vi "AFT Filter Signal (Real, PtByPt).vi"(7 "reset? (F)":bool, 8 "error in (no error)":errorcluster, 10 "x(n)":dbl, 11 "adaptive filter in":refnum<k20>) -> (0 "error out":errorcluster, 2 "y(n)":dbl, 3 "adaptive filter out":refnum<k20>)   [LabVIEW 2017, in "NI_AdaptiveFilter.lvlib"]
doc: "Filters an input signal with an adaptive filter point by point. You must use the least mean squares (LMS) or recursive least squares (RLS) algorithms to create the adaptive filter. Unlike the AFT Filter Signal and Update Coefficients VI, the AFT Filter Signal VI does not update the coefficients of the adaptive filter. Use the AFT Update Coefficients VI to update the filter coefficients. Wire data to the <B>x(n)</B> input to determine the polymorphic instance to use or manually select the instance. The data type of the adaptive filter that you wire to the <B>adaptive filter in</B> input must match the instance of the AFT Filter Signal VI."
uses:
  <vilib>/addons/Adaptive Filters/NI_AdaptiveFilter.lvlib
  <resource>/AdaptiveFilters.dll
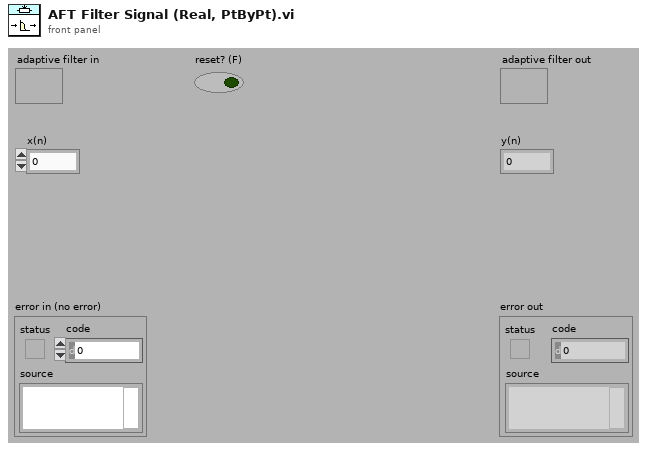
[diagram p1: front panel]
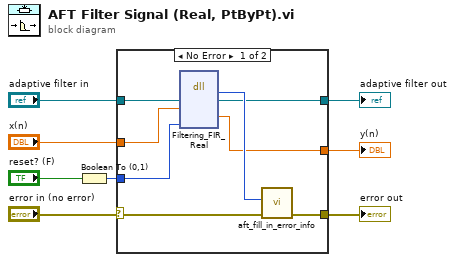
[diagram p0: block diagram]
diagram:
  n1 = Boolean To (0,1)(Boolean="reset? (F)") -> (0, 1=w5:i16)
  n2 = case shown="No Error" "error in (no error)" {
    selector: "error in (no error)" -> [w15 w18]
    tunnel: [w13 w18] -> w8
    tunnel: "adaptive filter in" -> [w10 w17]
    tunnel: "x(n)" -> [w16 _]
    tunnel: [w9 w17] -> w2
    tunnel: w5 -> [w12 _]
    tunnel: [w11 _] -> w1
    frame No Error {
      n3 = dll-call lib="C:/Program Files/National Instruments/LabVIEW 2017/resource/AdaptiveFilters.dll" fn="Filtering_FIR_Real" ("Complex Data Initialization")("pSession"=w10, "x"=w16, "reset"=w12) -> ("err"=w14:i32, "pSession"=w9:refnum<k20>, "y"=w11:dbl)  [unwired: 5 in, 3 out]
      n4 = call <vilib>:"aft_fill_in_error_info.vi"("error in"=w15, "status code"=w14) -> ("error out"=w13:errorcluster)  [unwired: 2 in, 7 out]
    }
    frame Error {
    }
  }
  "error out" <- w8
  "y(n)" <- w1
  "adaptive filter out" <- w2
